vi "edittest add missing fields to system.vi"(8 "error in (no error)":errorcluster, 9 "Fields":T2[](array[typedef]), 10 "sxSequenceId (\"\")":string, 11 "Connection Refnum":T1) -> (0 "error out":errorcluster, 3 "Connection Refnum":T1)   [LabVIEW 2011]
uses:
  server/database/Fields/Field Record.ctl
  server/database/Fields/Field DataTypes.ctl
  server/database/Fields/Field NextItem.ctl
  SI.LIB/ODBC/SQL Controls/Connection Refnum.ctl
  server/database/Fields/Field Order By.ctl
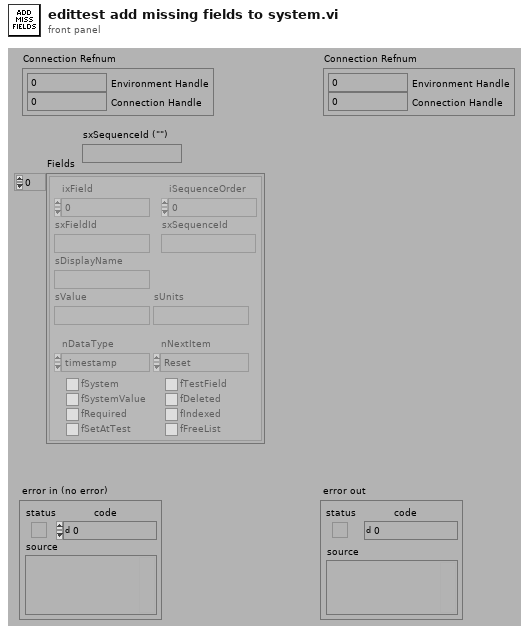
[diagram p1: front panel]
types:
  T1 = typedef "Connection Refnum.ctl" = cluster{"Environment Handle":i32, "Connection Handle":i32}
  T2 = typedef "Field Record.ctl" = cluster{"ixField":i32, "iSequenceOrder":i32, "sxFieldId":string, "sxSequenceId":string, "sDisplayName":string, "sValue":string, "sUnits":string, "nDataType":T3, "nNextItem":T4, "fSystem":bool, "fSystemValue":bool, "fRequired":bool, "fSetAtTest":bool, "fTestField":bool, "fDeleted":bool, "fIndexed":bool, "fFreeList":bool}
  T3 = typedef "Field DataTypes.ctl" = enum32{"text", "numeric", "list", "timestamp", "boolean"}
  T4 = typedef "Field NextItem.ctl" = enum32{"Reset", "Retain", "Auto-Increment"}
  T5 = typedef "Field Order By.ctl" = enum32{"sxSequenceId", "sxFieldId", "sDisplayName", "sValue", "fSetAtTest", "fRequired", "nNextItem"}
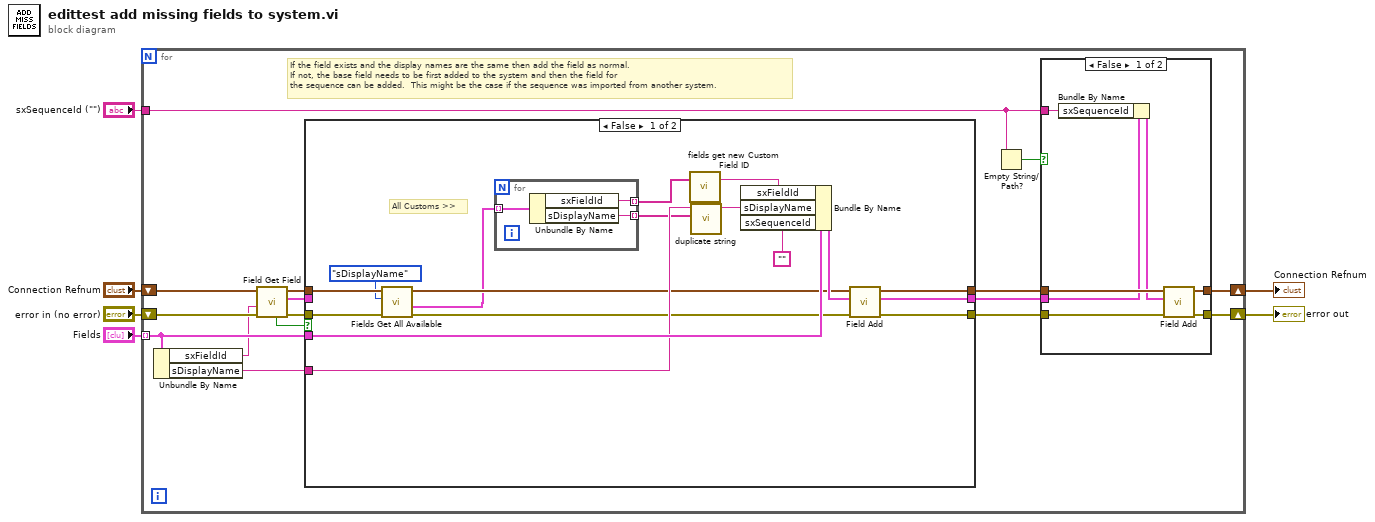
[diagram p0: block diagram]
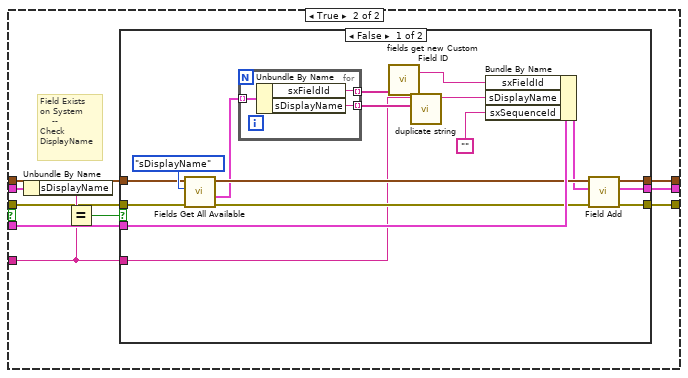
[diagram p3: hidden frame]
diagram:
  n1 = for {
    shift-right: [w21] -> w3
    shift-left: "Connection Refnum" -> [w18]
    shift-right: [w22] -> w2
    shift-left: "error in (no error)" -> [w19]
    tunnel: "Fields" -> [w20] mode=indexing
    tunnel: "sxSequenceId (\"\")" -> [w8]
    # "If the field exists and the display names are the same then add the field as normal.\nIf not, the base field needs to be first added to the system and then the field for\nthe sequence can be added.  This might be the case if the sequence was imported from another system."
    n2 = Unbundle By Name(w20) -> ("sxFieldId"=w17:string, "sDisplayName"=w12:string)
    n3 = call "Field Get Field.vi"("error in (no error)"=w19, "sFieldId or sDisplayName (\"\")"=w17, "Connection Refnum"=w18) -> ("error out"=w16:errorcluster, "Field"=w14:T2, "Connection Refnum"=w15:T1, "Data Present?"=w13:bool)  [unwired: 2 in, 3 out]
    n4 = case shown="False" w13 {
      tunnel: [w43 w51] -> w9
      tunnel: w20 -> [w45 w60]
      tunnel: w16 -> [w46 w55]
      tunnel: w15 -> [w47 w56]
      tunnel: w14 -> [_ w59]
      tunnel: w12 -> [w41 w54]
      tunnel: [w44 w53] -> w11
      tunnel: [w42 w52] -> w10
      frame False {
        # "All Customs >>"
        n5 = call "Fields Get All Available.vi"("error in (no error)"=w46, "Sort by (sxSequenceId)"=Field_Order_By."sDisplayName" ("Sort by (Sequence_ID)"), "Connection Refnum"=w47) -> ("error out"=w38:errorcluster, "Custom Fields"=w34:T2[], "Connection Refnum"=w39:T1)  [unwired: 2 in, 4 out]
        n6 = for {
          tunnel: w34 -> [w50] mode=indexing
          tunnel: [w49] -> w33 mode=indexing
          tunnel: [w48] -> w37 mode=indexing
          n7 = Unbundle By Name(w50) -> ("sxFieldId"=w49:string, "sDisplayName"=w48:string)
        }
        n8 = call "fields get new Custom Field ID.vi"("Existing Field IDs (empty)"=w33) -> ("Custom Field ID"=w32:string)  [unwired: 1 in, 1 out]
        n9 = call "duplicate string.vi"("Array of Strings"=w37, "String"=w41) -> ("Updated String"=w36:string)  [unwired: 9 out]
        n10 = Bundle By Name(cluster=w45, "sxFieldId"=w32, "sDisplayName"=w36, "sxSequenceId"="") -> (w43:T2)
        n11 = call "Field Add.vi"("error in (no error)"=w38, "Field Record"=w43, "Connection Refnum"=w39) -> ("error out"=w42:errorcluster, "Connection Refnum"=w44:T1)  [unwired: 1 in, 6 out]
      }
      frame True {
        # "Field Exists\non System\n    --\nCheck\nDisplayName"
        n12 = Unbundle By Name(w59) -> ("sDisplayName"=w58:string)
        n13 = Equal?(x=w58, y=w54) -> (x = y?=w57:bool)
        n14 = case shown="False" w57 {
          tunnel: [w64 w82] -> w51
          tunnel: w60 -> [w76 w82]
          tunnel: w56 -> [w72 w81]
          tunnel: w55 -> [w73 w80]
          tunnel: w54 -> [w68 _]
          tunnel: [w66 w81] -> w53
          tunnel: [w65 w80] -> w52
          frame False {
            n15 = call "Fields Get All Available.vi"("error in (no error)"=w73, "Sort by (sxSequenceId)"=Field_Order_By."sDisplayName" ("Sort by (Sequence_ID)"), "Connection Refnum"=w72) -> ("error out"=w70:errorcluster, "Custom Fields"=w63:T2[], "Connection Refnum"=w71:T1)  [unwired: 2 in, 4 out]
            n16 = for {
              tunnel: w63 -> [w79] mode=indexing
              tunnel: [w78] -> w62 mode=indexing
              tunnel: [w77] -> w69 mode=indexing
              n17 = Unbundle By Name(w79) -> ("sxFieldId"=w78:string, "sDisplayName"=w77:string)
            }
            n18 = call "fields get new Custom Field ID.vi"("Existing Field IDs (empty)"=w62) -> ("Custom Field ID"=w61:string)  [unwired: 1 in, 1 out]
            n19 = call "duplicate string.vi"("Array of Strings"=w69, "String"=w68) -> ("Updated String"=w67:string)  [unwired: 9 out]
            n20 = Bundle By Name(cluster=w76, "sxFieldId"=w61, "sDisplayName"=w67, "sxSequenceId"="") -> (w64:T2)
            n21 = call "Field Add.vi"("error in (no error)"=w70, "Field Record"=w64, "Connection Refnum"=w71) -> ("error out"=w65:errorcluster, "Connection Refnum"=w66:T1)  [unwired: 1 in, 6 out]
          }
          frame True {
          }
        }
      }
    }
    n22 = Empty String/Path?(string/path=w8) -> (empty?=w7:bool)
    n23 = case shown="False" w7 {
      tunnel: [w29 w30] -> w22
      tunnel: [w28 w31] -> w21
      tunnel: w11 -> [w27 w31]
      tunnel: w10 -> [w26 w30]
      tunnel: w9 -> [w24 _]
      tunnel: w8 -> [w23 _]
      frame False {
        n24 = Bundle By Name(cluster=w24, "sxSequenceId"=w23) -> (w25:T2)
        n25 = call "Field Add.vi"("error in (no error)"=w26, "Field Record"=w25, "Connection Refnum"=w27) -> ("error out"=w29:errorcluster, "Connection Refnum"=w28:T1)  [unwired: 1 in, 6 out]
      }
      frame True {
      }
    }
  }
  "error out" <- w2
  "Connection Refnum" <- w3
